vi "PropertyListCheckSelection.vi"(10 "Selectrion in":string[](array[string]), 11 "All Tags":string[](array[string])) -> (2 "Children removed":set{string}(c389), 3 "Selection out":string[](array[string]))   [LabVIEW 2020, in "VIPropertyPicker.lvlib"]
uses:
  VIPropertyPicker.lvlib
  e54d4e2b-e6f6-488c-9e70-f23a01a6a315.vi
  47fcd4a0-3797-4089-abe1-4a3053e93a78.vi
  8e9b9a24-754c-46f4-a281-83c5f9bd1ac6.vi
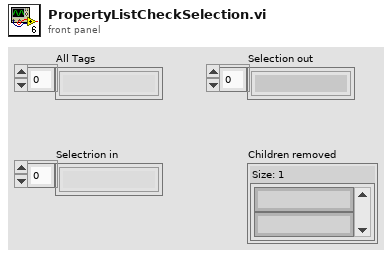
[diagram p1: front panel]
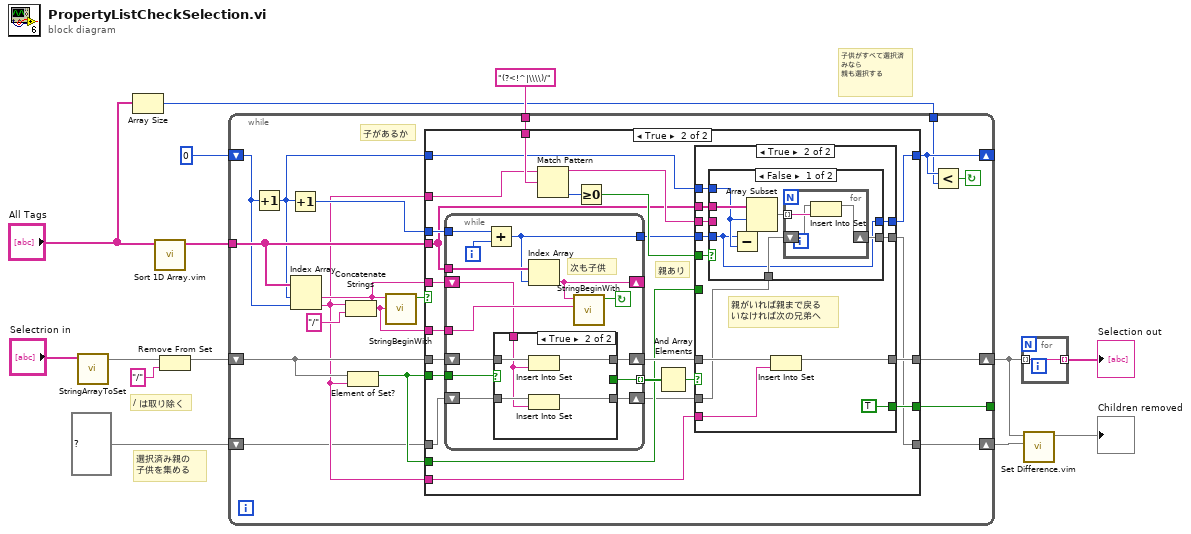
[diagram p0: block diagram]
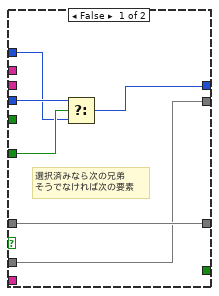
[diagram p3: hidden frame]
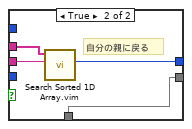
[diagram p4: hidden frame]
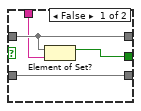
[diagram p5: hidden frame]
diagram:
  # "選択済み親の\n子供を集める"
  # "/ は取り除く"
  # "子供がすべて選択済みなら\n親も選択する"
  n1 = call "StringArrayToSet.vi"("String Array"="Selectrion in") -> ("Set"=w11:set{string})  [unwired: 10 in]
  n2 = Array Size(array="All Tags") -> (size(s)=w7:i32)
  n3 = call "Sort 1D Array.vim"("unsorted array"="All Tags") -> ("sorted array"=w13:string[])  [unwired: 10 in]
  n4 = Remove From Set(10:"/" ("element"), 11:w11) -> (3:w10:set{string})  [unwired: 1 out]
  n5 = while {
    shift-right: [w17] -> _
    shift-left: 0 -> [w23]
    tunnel: w13 -> [w31]
    shift-right: [w26] -> w5
    shift-left: w10 -> [w28]
    tunnel: [w25] -> _
    tunnel: "(?<!^|\\\\)/" ("regular expression") -> [w22]
    shift-right: [w18] -> w6
    shift-left: set{string} {} ("set out") -> [w19]
    tunnel: w7 -> [w16]
    stop <- w15 continue-if-true
    # "子があるか"
    n6 = Increment(x=w23) -> (x+1=w24:i32)
    n7 = Increment(x=w24) -> (x+1=w29:i32)
    n8 = Index Array(array=w31, index #1=w24, index #2=w23) -> (element #1=w27:string, element #2=w21:string)
    n9 = Concatenate Strings(w21, "/" ("string")) -> (w30:string)
    n10 = Element of Set?(10:w21, 11:w28) -> (3:w20:bool)
    n11 = call "StringBeginWith.vi"("Begin With"=w30, "String"=w27) -> ("StringBeginWith"=w32:bool)  [unwired: 9 in]
    n12 = case shown="True" w32 {
      tunnel: w29 -> [_ w60]
      tunnel: w31 -> [_ w44]
      tunnel: w30 -> [_ w59]
      tunnel: w20 -> [_ w58]
      tunnel: w28 -> [w36 w57]
      tunnel: w27 -> [_ w56]
      tunnel: [w36 w52] -> w26
      tunnel: w21 -> [_ w51]
      tunnel: [_ w50] -> w25
      tunnel: w24 -> [w35 w40]
      tunnel: [w35 w43] -> w17
      tunnel: w22 -> [_ w49]
      tunnel: w21 -> [_ w48]
      tunnel: w20 -> [_ w41]
      tunnel: w19 -> [w34 w39]
      tunnel: [w34 w37] -> w18
      frame False {
      }
      frame True {
        # "親あり"
        n13 = while {
          tunnel: w60 -> [w106]
          tunnel: w44 -> [w104]
          tunnel: w59 -> [w103]
          tunnel: w58 -> [w98]
          shift-right: [w100] -> _
          shift-left: w56 -> [w99]
          tunnel: [w96] -> w55 mode=indexing
          tunnel: [w95] -> w42
          shift-right: [w97] -> w53
          shift-left: w57 -> [w101]
          shift-right: [w93] -> w38
          shift-left: w39 -> [w94]
          i -> [w105]
          stop <- w102 continue-if-true
          # "次も子供"
          n14 = Add(x=w106, y=w105) -> (x+y=w95:i32)
          n15 = case shown="True" w98 {
            tunnel: w101 -> [w110 w115]
            tunnel: w99 -> [w109 w112]
            tunnel: [w110 w114] -> w97
            tunnel: [w108 _] -> w96
            tunnel: w94 -> [w107 w113]
            tunnel: [w107 w111] -> w93
            frame False {
              n16 = Element of Set?(10:w109, 11:w110) -> (3:w108:bool)
            }
            frame True {
              n17 = Insert Into Set(10:w112, 11:w115) -> (3:w114:set{string})  [unwired: 1 out]
              n18 = Insert Into Set(10:w112, 11:w113) -> (3:w111:set{string})  [unwired: 1 out]
            }
          }
          n19 = Index Array(array=w104, index=w95) -> (element=w100:string)
          n20 = call "StringBeginWith.vi"("Begin With"=w103, "String"=w100) -> ("StringBeginWith"=w102:bool)  [unwired: 9 in]
        }
        n21 = Match Pattern(string=w48, regular expression=w49) -> (before substring=w45:string, offset past match=w47:i32)  [unwired: 1 in, 2 out]
        n22 = Greater Or Equal To 0?(x=w47) -> (x >= 0?=w46:bool)
        n23 = And Array Elements(Boolean array=w55) -> (logical AND=w54:bool)
        n24 = case shown="True" w54 {
          tunnel: w53 -> [w66 w78]
          tunnel: [w66 w77] -> w52
          tunnel: w51 -> [_ w75]
          tunnel: [_ TRUE] -> w50
          tunnel: w46 -> [_ w74]
          tunnel: w45 -> [_ w73]
          tunnel: w44 -> [_ w72]
          tunnel: [w62 w71] -> w43
          tunnel: w42 -> [w64 w70]
          tunnel: w41 -> [w65 _]
          tunnel: w40 -> [w63 w69]
          tunnel: w38 -> [w61 w68]
          tunnel: [w61 w67] -> w37
          frame False {
            # "選択済みなら次の兄弟\nそうでなければ次の要素"
            n25 = Select(t=w64, s=w65, f=w63) -> (s? t:f=w62:i32)
          }
          frame True {
            # "親がいれば親まで戻る\nいなければ次の兄弟へ"
            # "子供が"
            n26 = case shown="False" w74 {
              tunnel: w73 -> [_ w92]
              tunnel: w72 -> [w85 w91]
              tunnel: [w79 w90] -> w71
              tunnel: w70 -> [w79 _]
              tunnel: w69 -> [w84 _]
              tunnel: w68 -> [w81 w89]
              tunnel: [w80 w89] -> w67
              frame False {
                n27 = Subtract(x=w79, y=w84) -> (x-y=w83:i32)
                n28 = Array Subset(array=w85, index=w84, length=w83) -> (w82:string[])
                n29 = for {
                  tunnel: w82 -> [w88] mode=indexing
                  shift-right: [w86] -> w80
                  shift-left: w81 -> [w87]
                  n30 = Insert Into Set(10:w88, 11:w87) -> (3:w86:set{string})  [unwired: 1 out]
                }
              }
              frame True {
                # "自分の親に戻る"
                n31 = call "Search Sorted 1D Array.vim"("element"=w92, "sorted 1D array"=w91) -> ("nearest index"=w90:i32)  [unwired: 8 in, 1 out]
              }
            }
            n32 = Insert Into Set(10:w75, 11:w78) -> (3:w77:set{string})  [unwired: 1 out]
          }
        }
      }
    }
    n33 = Less?(x=w17, y=w16) -> (x < y?=w15:bool)
  }
  n34 = for {
    tunnel: [w116] -> w1 mode=indexing
    tunnel: w5 -> [w116] mode=indexing
  }
  "Selection out" <- w1
  n35 = call "Set Difference.vim"("set 2"=w6, "set 1"=w5) -> ("difference"=→"Children removed":set{string})  [unwired: 9 in]
